vi "InTake Process.vi"(0 "error in":errorcluster) -> ()   [LabVIEW 2013]
uses:
  InTake Global Data.vi
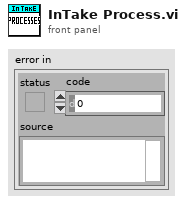
[diagram p1: front panel]
types:
  T1 = typedef "WPI_SolenoidValue.ctl" = enum16{"Off", "On", "Forward", "Reverse"}
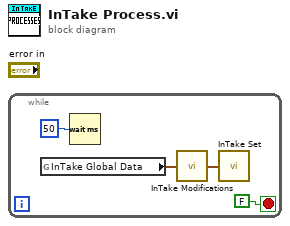
[diagram p0: block diagram]
diagram:
  n1 = while {
    stop <- FALSE stop-if-true
    n2 = global read "InTake Global Data.vi" "InTake Global Data"() -> (w2:cluster{"TakeBall":dbl, "MoveArm":T1})
    n3 = Wait (ms)(milliseconds to wait=u32 50) -> ()  [unwired: 1 out]
    n4 = call "InTake Modifications.vi"("InTake Global Data In"=w2) -> ("InTake Global Data Out"=w1:cluster{"TakeBall":dbl, "MoveArm":T1})
    n5 = call "InTake Set.vi"("InTake"=w1) -> ()
  }
